vi "Angle evaluator.vi"(9 "Position Az":dbl, 10 "Position Bz":dbl, 11 "Position Cz":dbl) -> (2 "beta (z-y angle)":dbl, 3 "alpha (z-x angle)":dbl)   [LabVIEW 2017]
uses:
  <userlib>/_MGI/Numeric/Coercion/MGI Radians to Degrees/MGI Radians to Degrees DBL.vi
panel:
  # "C"
  # "O"
  # "A"
  # "B"
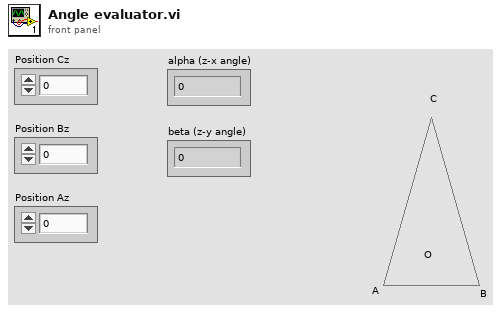
[diagram p1: front panel]
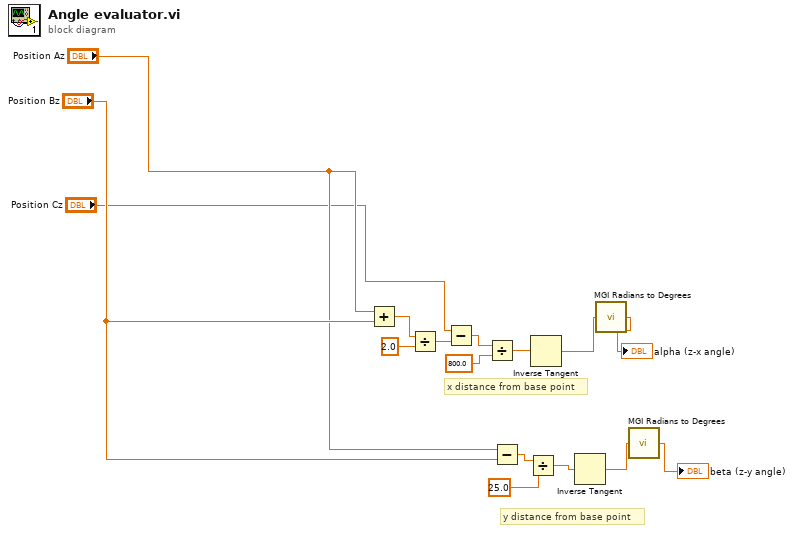
[diagram p0: block diagram]
diagram:
  # "y distance from base point"
  # "x distance from base point"
  n1 = Add(x="Position Az", y="Position Bz") -> (x+y=w6:dbl)
  n2 = Divide(x=w6, y=2.0) -> (x/y=w8:dbl)
  n3 = Subtract(x="Position Cz", y=w8) -> (x-y=w10:dbl)
  n4 = Divide(x=w10, y=800.0) -> (x/y=w11:dbl)
  n5 = Subtract(x="Position Az", y="Position Bz") -> (x-y=w14:dbl)
  n6 = Divide(x=w14, y=25.0) -> (x/y=w15:dbl)
  n7 = Inverse Tangent(1:w11) -> (0:w4:dbl)
  n8 = Inverse Tangent(1:w15) -> (0:w3:dbl)
  n9 = call-poly <userlib>:"MGI Radians to Degrees.vi"("Radians"=w4) -> ("Degrees"=→"alpha (z-x angle)":dbl)
  n10 = call-poly <userlib>:"MGI Radians to Degrees.vi"("Radians"=w3) -> ("Degrees"=→"beta (z-y angle)":dbl)
